vi "MCB2300 PWM Conflict ProjectAttrValidator.vi"(5 "Ctl Refnum":refnum<vi>, 7 "IO Name (original)":string, 9 "IO Channel Number":i32(ring) items=["0", "1", "2", "3", "4", "5", "6", "7", "8", "9", "10", "11", "12", "13", "14", "15", "16", "17", "18", "19", "20", "21", "22", "23", "24", "25", "26", "27", "28", "29", "30", "31", "32", "33", "34", "35", "36", "37", "38", "39", "40", "41", "42", "43", "44", "45", "46", "47", "48", "49", "50", "51", "52", "53", "54", "55", "56", "57", "58", "59", "60", "61", "62", "63", "64", "65", "66", "67", "68", "69", "70", "71", "72", "73", "74", "75", "76", "77", "78", "79", "80", "81", "82", "83", "84", "85", "86", "87", "88", "89", "90", "91", "92", "93", "94", "95", "96", "97", "98", "99", "100", "101", "102", "103", "104", "105", "106", "107", "108", "109", "110", "111", "112", "113", "114", "115", "116", "117", "118", "119", "120", "121", "122", "123", "124", "125", "126", "127", "128", "129", "130", "131", "132", "133", "134", "135", "136", ""], 11 "Project Attributes":T1={"Offset%"=0, "Double edge?"=FALSE, "Polarity"=FALSE, "Frequency"=1000, "Programmable Pin Connections"=0} {"Programmable Pin Connections" items=["PWM0 uses pin P2.0. You can not use PWM0 and pin P2.0 in the same project.", "PWM1 uses pin P2.1. You can not use PWM1 and pin P2.1 in the same project.", "PWM2 uses pin P2.2. You can not use PWM2 and pin P2.2 in the same project.", "PWM3 uses pin P2.3. You can not use PWM3 and pin P2.3 in the same project.", "PWM4 uses pin P2.4. You can not use PWM4 and pin P2.4 in the same project.", "PWM5 uses pin P2.5. You can not use PWM5 and pin P2.5 in the same project."]}) -> (3 "Valid?":bool)   [LabVIEW 2011]
uses:
  <vilib>/Embedded/ARM/MCB2300/MCB2300_PWM_Conflicts_PrjAttr.ctl
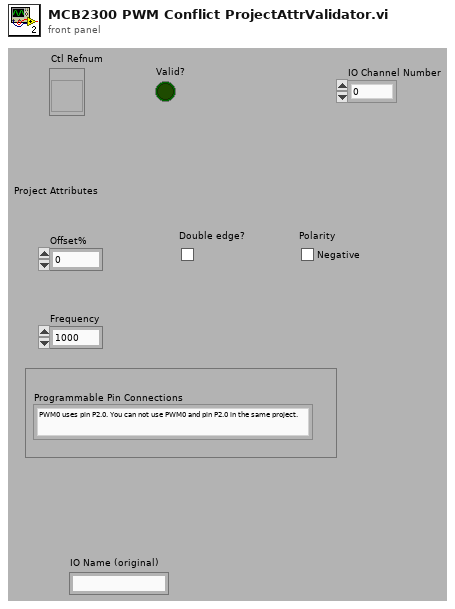
[diagram p1: front panel]
types:
  T1 = typedef "MCB2300_PWM_Conflicts_PrjAttr.ctl" = cluster{"Offset%":u8, "Double edge?":bool, "Polarity":bool, "Frequency":u32, "Programmable Pin Connections":u16}
  T2 = cluster{"Offset%":u8, "Double edge?":bool, "Polarity":bool, "Frequency":u32, "Programmable Pin Connections":u16}
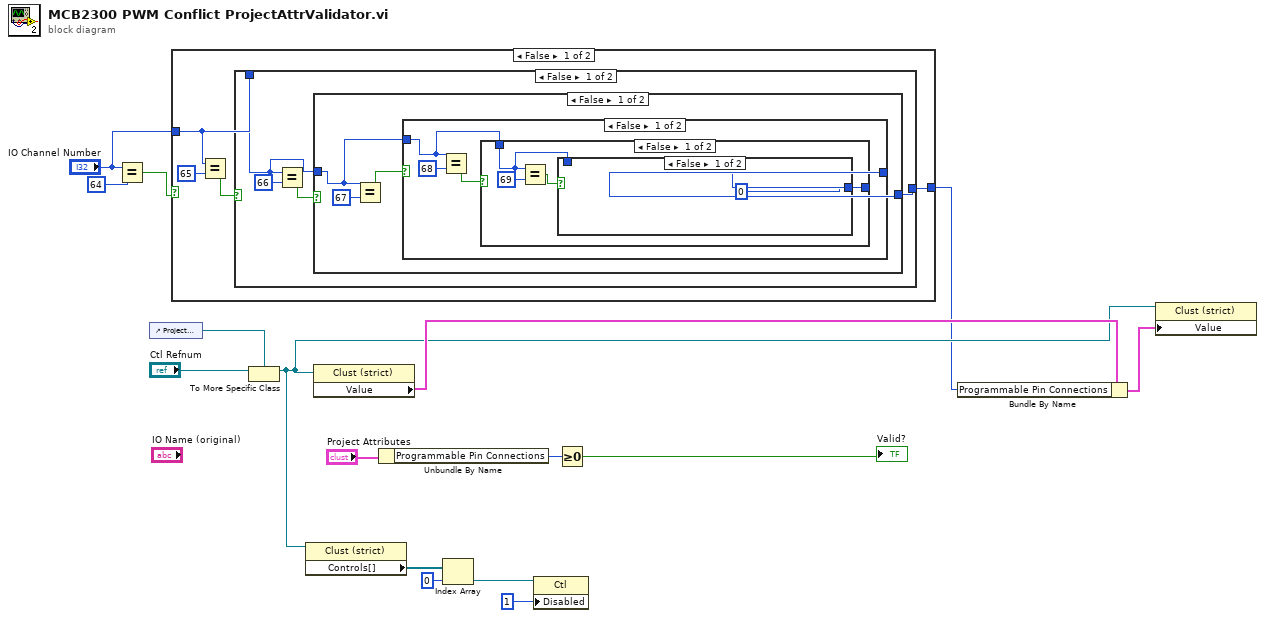
[diagram p0: block diagram]
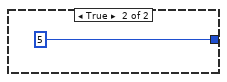
[diagram p2: hidden frame]
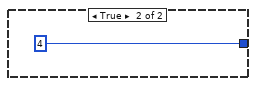
[diagram p3: hidden frame]
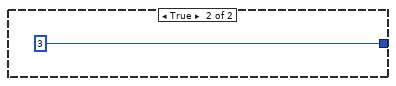
[diagram p4: hidden frame]
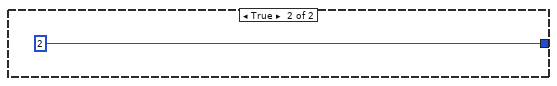
[diagram p5: hidden frame]
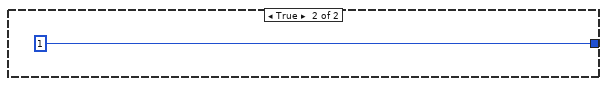
[diagram p6: hidden frame]
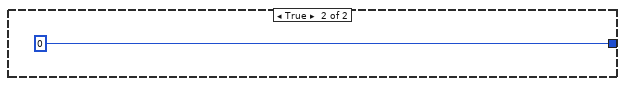
[diagram p7: hidden frame]
diagram:
  n1 = Equal?(x="IO Channel Number", y=64) -> (x = y?=w2:bool)
  n2 = control-ref of="Project Attributes"() -> (w15:refnum<vi>)
  n3 = case shown="False" w2 {
    tunnel: [w18 0] -> w3
    tunnel: "IO Channel Number" -> [w17 _]
    frame False {
      n4 = Equal?(x=w17, y=65) -> (x = y?=w19:bool)
      n5 = case shown="False" w19 {
        tunnel: [w22 1] -> w18
        tunnel: w17 -> [w21 _]
        frame False {
          n6 = Equal?(x=w21, y=66) -> (x = y?=w23:bool)
          n7 = case shown="False" w23 {
            tunnel: [w26 2] -> w22
            tunnel: w21 -> [w25 _]
            frame False {
              n8 = Equal?(x=w25, y=67) -> (x = y?=w27:bool)
              n9 = case shown="False" w27 {
                tunnel: [w30 3] -> w26
                tunnel: w25 -> [w29 _]
                frame False {
                  n10 = Equal?(x=w29, y=68) -> (x = y?=w31:bool)
                  n11 = case shown="False" w31 {
                    tunnel: [w34 4] -> w30
                    tunnel: w29 -> [w33 _]
                    frame False {
                      n12 = Equal?(x=w33, y=69) -> (x = y?=w35:bool)
                      n13 = case shown="False" w35 {
                        tunnel: [0 5] -> w34
                        tunnel: w33 -> [_ _]
                        frame False {
                        }
                        frame True {
                        }
                      }
                    }
                    frame True {
                    }
                  }
                }
                frame True {
                }
              }
            }
            frame True {
            }
          }
        }
        frame True {
        }
      }
    }
    frame True {
    }
  }
  n14 = To More Specific Class(target class=w15, reference="Ctl Refnum") -> (specific class reference=w5:refnum<vi>)  [unwired: 1 in, 1 out]
  n15 = property class="Clust (strict)"(reference=w5) -> ("Controls[]"=w12:refnum<vi>[])  [unwired: 1 in, 2 out]
  n16 = property class="Clust (strict)"(reference=w5) -> ("Value"=w14:T2)  [unwired: 1 in, 2 out]
  n17 = Unbundle By Name("Project Attributes") -> ("Programmable Pin Connections"=w7:u16)
  n18 = Index Array(array=w12, index=0) -> (element=w10:refnum<vi>)
  n19 = property class="Ctl"(reference=w10, "Disabled"=u8 1) -> ()  [unwired: 1 in, 2 out]
  n20 = Greater Or Equal To 0?(x=w7) -> (x >= 0?=→"Valid?":bool)
  n21 = Bundle By Name(cluster=w14, "Programmable Pin Connections"=w3) -> (w13:T2)
  n22 = property class="Clust (strict)"(reference=w5, "Value"=w13) -> ()  [unwired: 1 in, 2 out]
